vi "利用海伦公式计算三角形面积.vi"(1 "c":dbl, 2 "b":dbl, 3 "a":dbl) -> (0 "Area":dbl)   [LabVIEW 2012, in "几何工具.lvlib"]
doc: "功能：\n\n利用三角形三个边长（a b c）计算三角形的面积。\n\n公式：\n\n1、s=(a+b+c)/2\n2、A=sqrt(s*(s-a)*(s-b)*(s-c))"
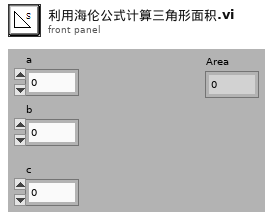
[diagram p1: front panel]
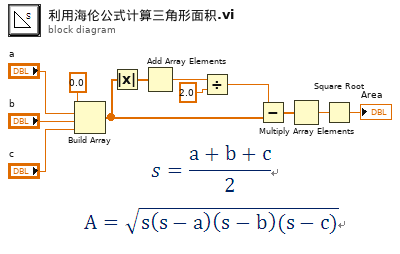
[diagram p0: block diagram]
diagram:
  n1 = Build Array(0.0 ("元素"), "a", "b", "c") -> (w7:dbl[])
  n2 = Absolute Value(x=w7) -> (abs(x)=w9:dbl[])
  n3 = Add Array Elements(numeric array=w9) -> (sum=w4:dbl)
  n4 = Divide(x=w4, y=2.0 ("a")) -> (x/y=w3:dbl)
  n5 = Subtract(x=w3, y=w7) -> (x-y=w6:dbl[])
  n6 = Multiply Array Elements(1:w6) -> (0:w1:dbl)
  n7 = Square Root(x=w1) -> (sqrt(x)=→"Area":dbl)
